vi "Get RT Configuration.vi"(8 "error in (no error)":errorcluster, 11 "Device Reference in":T1 format="%.0x") -> (0 "error out":errorcluster, 3 "RT Config":T2 {"Config"."Industrial Settings"."Write Refs"."Data Reference" format="%.0x"; "Config"."Industrial Settings"."Read Refs"."Data Reference" format="%.0x"; "Config"."PID Settings"."Read Refs"."Data Reference" format="%.0x"; "Config"."PID Settings"."Write Refs"."Data Reference" format="%.0x"})   [LabVIEW 2019, in "Control Addon Engine.lvlib"]
uses:
  Control Addon Engine.lvlib
  Types/RT Configuration.ctl
  Shared/Types/Gain Schedule.ctl
  Shared/Types/Compiled Settings.ctl
  Shared/Types/Compiled PID Settings.ctl
  <vilib>/NI VeriStand/Custom Device API/Block Data Reference.ctl
  <vilib>/NI VeriStand/Custom Device API/Data Reference.ctl
  Shared/Types/Compiled Industrial Settings.ctl
  Shared/Types/Compiled Industrial Parameters.ctl
  <vilib>/NI VeriStand/Custom Device API/Custom Device Item Ref.ctl
  Shared/Constants.vi
  <vilib>/NI VeriStand/Custom Device API/Get Item Property (Variant).vi
  Shared/Control Addon Shared.lvlib
  <vilib>/NI VeriStand/Custom Device API/Custom Device API.lvlib
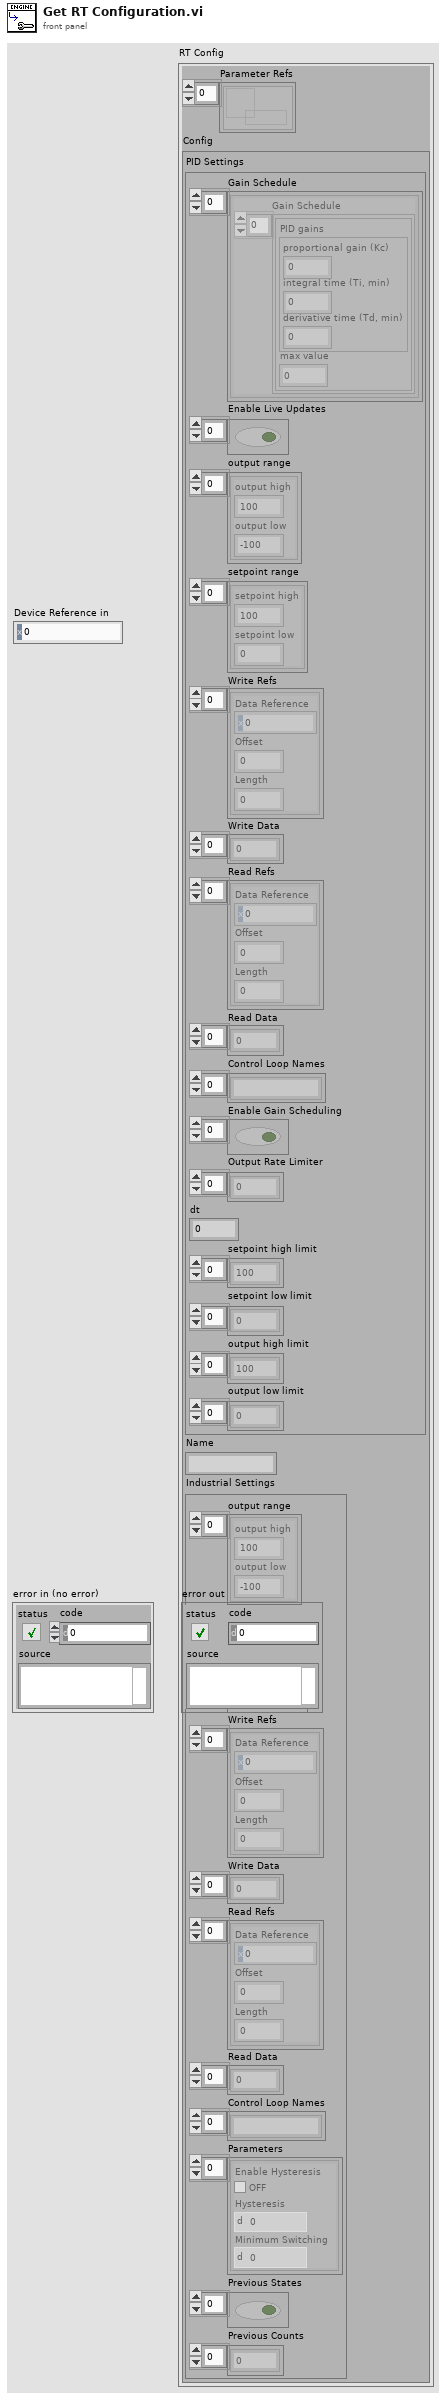
[diagram p1: front panel]
types:
  T1 = typedef "Custom Device API.lvlib/Custom Device Item Ref.ctl" = u64
  T2 = typedef "Control Addon Engine.lvlib/RT Configuration.ctl" = cluster{"Parameter Refs":refnum<data-value>[], "Config":T3}
  T3 = typedef "Control Addon Shared.lvlib/Compiled Settings.ctl" = cluster{"PID Settings":T4, "Name":string, "Industrial Settings":T8}
  T4 = typedef "Control Addon Shared.lvlib/Compiled PID Settings.ctl" = cluster{"Gain Schedule":T5[], "Enable Live Updates":bool[], "output range":cluster{"output high":dbl, "output low":dbl}[], "setpoint range":cluster{"setpoint high":dbl, "setpoint low":dbl}[], "Write Refs":T6[], "Write Data":dbl[], "Read Refs":T6[], "Read Data":dbl[], "Control Loop Names":string[], "Enable Gain Scheduling":bool[], "Output Rate Limiter":dbl[], "dt":dbl, "setpoint high limit":dbl[], "setpoint low limit":dbl[], "output high limit":dbl[], "output low limit":dbl[]}
  T5 = typedef "Control Addon Shared.lvlib/Gain Schedule.ctl" = cluster{"Gain Schedule":cluster{"PID gains":cluster{"proportional gain (Kc)":dbl, "integral time (Ti, min)":dbl, "derivative time (Td, min)":dbl}, "max value":dbl}[]}
  T6 = typedef "Custom Device API.lvlib/Block Data Reference.ctl" = cluster{"Data Reference":T7, "Offset":u64, "Length":u64}
  T7 = typedef "Custom Device API.lvlib/Data Reference.ctl" = i32
  T8 = typedef "Control Addon Shared.lvlib/Compiled Industrial Settings.ctl" = cluster{"output range":cluster{"output high":dbl, "output low":dbl}[], "setpoint range":cluster{"setpoint high":dbl, "setpoint low":dbl}[], "Write Refs":T6[], "Write Data":dbl[], "Read Refs":T6[], "Read Data":dbl[], "Control Loop Names":string[], "Parameters":T9[], "Previous States":bool[], "Previous Counts":u64[]}
  T9 = typedef "Control Addon Shared.lvlib/Compiled Industrial Parameters.ctl" = cluster{"Enable Hysteresis":bool, "Hysteresis":dbl, "Minimum Switching":u64}
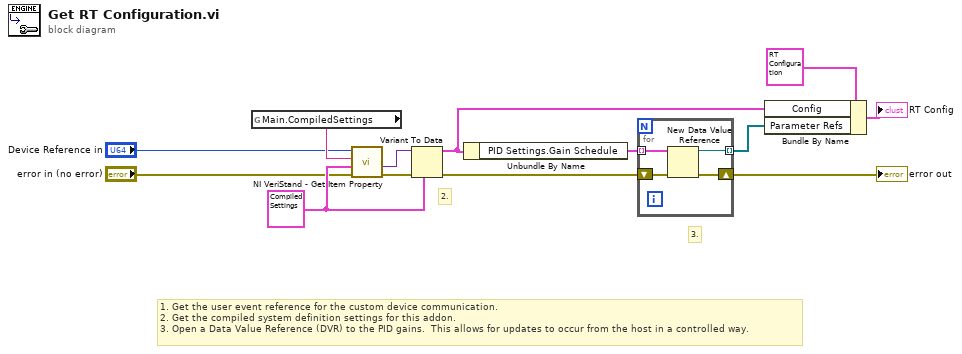
[diagram p0: block diagram]
diagram:
  w6 = T3 {"PID Settings"={"Gain Schedule"=[], "Enable Live Updates"=[], "output range"=[], "setpoint range"=[], "Write Refs"=[], "Write Data"=[], "Read Refs"=[], "Read Data"=[], "Control Loop Names"=[], "Enable Gain Scheduling"=[], "Output Rate Limiter"=[], "dt"=0.0, "setpoint high limit"=[], "setpoint low limit"=[], "output high limit"=[], "output low limit"=[]}, "Name"="", "Industrial Settings"={"output range"=[], "setpoint range"=[], "Write Refs"=[], "Write Data"=[], "Read Refs"=[], "Read Data"=[], "Control Loop Names"=[], "Parameters"=[], "Previous States"=[], "Previous Counts"=[]}} ("Cluster")
  # "1. Get the user event reference for the custom device communication.\n2. Get the compiled system definition settings for this addon.\n3. Open a Data Value Reference (DVR) to the PID gains.  This allows for updates to occur from the host in a controlled way."
  # "3."
  # "2."
  n1 = global read "Constants.vi" "Main.CompiledSettings"() -> (w3:string)
  n2 = call-poly <vilib>:"NI VeriStand - Get Item Property.vi"("error in (no error)"="error in (no error)", "Default Value"=w6, "Property Name"=w3, "Item Ref in"="Device Reference in") -> ("error out"=w4:errorcluster, "Value"=w5:variant)  [unwired: 4 in, 2 out]
  n3 = Variant To Data(error in=w4, type=w6, Variant=w5) -> (data=w13:T3, error out=w7:errorcluster)
  n4 = Unbundle By Name(w13) -> ("PID Settings.Gain Schedule"=w9:T5[])
  n5 = for {
    tunnel: w9 -> [w17] mode=indexing
    shift-right: [w15] -> w8
    shift-left: w7 -> [w16]
    tunnel: [w14] -> w10 mode=indexing
    n6 = New Data Value Reference(data value=w17, error in=w16) -> (data value reference=w14:refnum<data-value>, error out=w15:errorcluster)
  }
  "error out" <- w8
  n7 = Bundle By Name(cluster=T2 {"Parameter Refs"=[], "Config"={"PID Settings"={"Gain Schedule"=[], "Enable Live Updates"=[], "output range"=[], "setpoint range"=[], "Write Refs"=[], "Write Data"=[], "Read Refs"=[], "Read Data"=[], "Control Loop Names"=[], "Enable Gain Scheduling"=[], "Output Rate Limiter"=[], "dt"=0.0, "setpoint high limit"=[], "setpoint low limit"=[], "output high limit"=[], "output low limit"=[]}, "Name"="", "Industrial Settings"={"output range"=[], "setpoint range"=[], "Write Refs"=[], "Write Data"=[], "Read Refs"=[], "Read Data"=[], "Control Loop Names"=[], "Parameters"=[], "Previous States"=[], "Previous Counts"=[]}}} ("data"), "Config"=w13, "Parameter Refs"=w10) -> (→"RT Config":T2)
